vi "ADC.vi"() -> ()   [LabVIEW 2013]
uses:
  <vilib>/Utility/file.llb/Write To Spreadsheet File (DBL).vi
panel:
  out "Відповідне значення температури з урахуванням коеф. А":dbl
  in  "А коеф.":dbl=0.00784
  out "I А":dbl
  out "Rx оМ з урахуванням\n томпер. коеф А.":dbl
  out "Rx оМ":dbl
  out "Uadc В":dbl
  in  "А коеф.":dbl=0.0079
  in  "Path":path=path "C:/Temp_Do_msp430g2231/USB_PC_Config/first.csv"
  out "Відповідне значення температури":dbl
  in  "Опір при температурі ххС":dbl=1000.0
  in  "Значення Т ххС":dbl=25.0
  in  "АЦП розрядність":dbl=1024.0
  in  "Vcc":dbl=3.3
  in  "R0":dbl=1200.0
  out "Thermometer":dbl(slide) scale=-55.0..155.0
  out "Посилка":i32
  in  "stop":bool
  out "відповідний Числовий тип":dbl
  out "Отриманий текст":string
  in  "Вибір порта для\n отримання даних":refnum<visa-resource-name>
  # "Налаштування  для  датчика"
  # "Отримані дані"
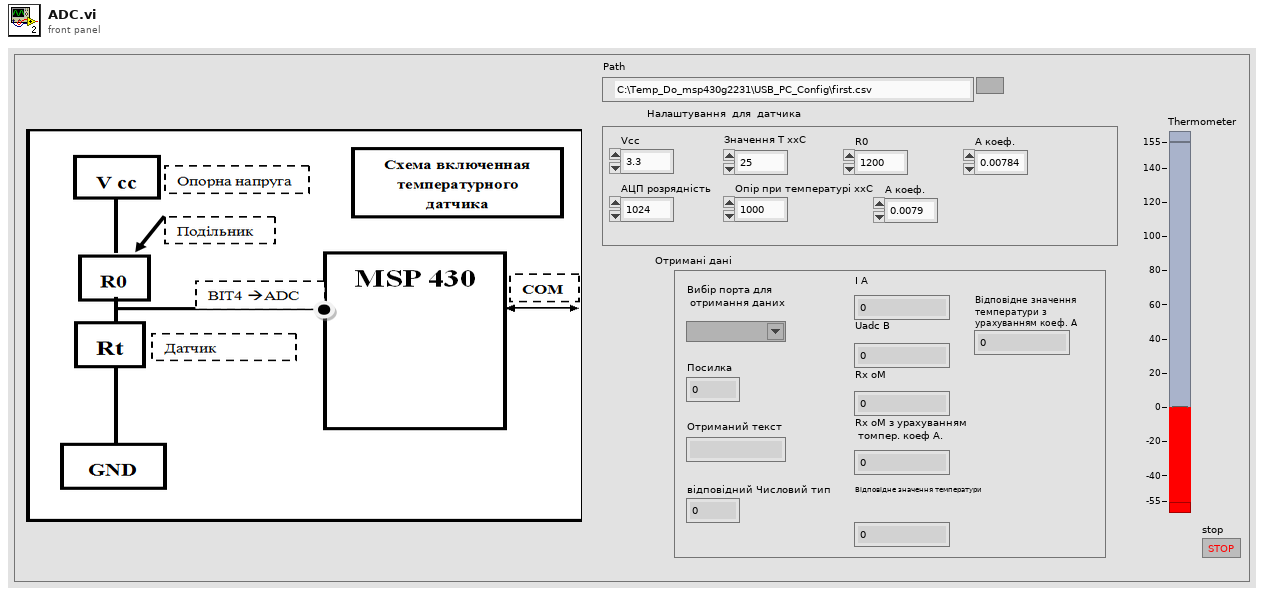
[diagram p1: front panel]
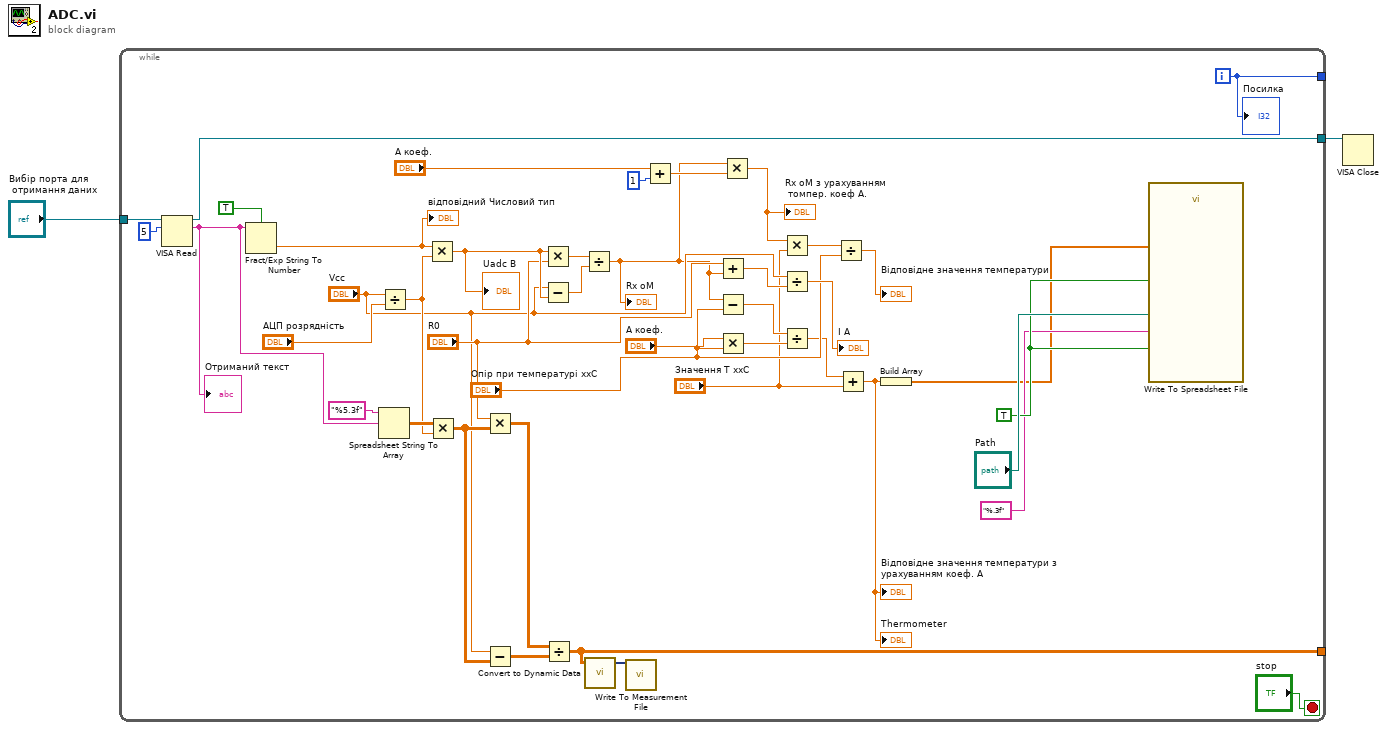
[diagram p0: block diagram]
diagram:
  n1 = while {
    tunnel: "Вибір порта для\n отримання даних" -> [w44]
    tunnel: [w25] -> _
    tunnel: [w28] -> _
    tunnel: [w32] -> w1
    i -> [w25]
    stop <- "stop" stop-if-true
    w27 = TRUE
    n2 = VISA Read(VISA resource name=w44, byte count=u32 5) -> (VISA resource name out=w32:refnum<visa-resource-name>, read buffer=w40:string)  [unwired: 1 in, 2 out]
    "Отриманий текст" <- w40
    n3 = Fract/Exp String To Number(use system decimal point (T)=TRUE, string=w40) -> (number=w33:dbl)  [unwired: 2 in, 1 out]
    "відповідний Числовий тип" <- w33
    n4 = Spreadsheet String To Array(format string="%5.3f", spreadsheet string=w40) -> (array=w34:dbl[][])  [unwired: 2 in]
    n5 = Divide(x="Vcc", y="АЦП розрядність") -> (x/y=w30:dbl)
    n6 = Multiply(x=w33, y=w30) -> (x*y=w19:dbl)
    "Uadc В" <- w19
    n7 = Multiply(x=w34, y=w30) -> (x*y=w39:dbl[][])
    n8 = Multiply(x="R0", y=w39) -> (x*y=w38:dbl[][])
    n9 = Subtract(x="Vcc", y=w39) -> (x-y=w37:dbl[][])
    n10 = Multiply(x=w19, y="R0") -> (x*y=w20:dbl)
    n11 = Subtract(x="Vcc", y=w19) -> (x-y=w21:dbl)
    n12 = Divide(x=w38, y=w37) -> (x/y=w28:dbl[][])
    n13 = Divide(x=w20, y=w21) -> (x/y=w10:dbl)
    "Rx оМ" <- w10
    n14 = call "Convert to Dynamic Data"("2D Array"=w28) -> ("Dynamic Data Type"=w35:dynamicdata)  [unwired: 3 in]
    n15 = call "Write To Measurement File"("Signals"=w35) -> ()  [unwired: 16 in, 3 out]
    n16 = Add(x="А коеф.", y=1) -> (x+y=w18:dbl)
    n17 = Add(x="R0", y=w10) -> (x+y=w16:dbl)
    n18 = Subtract(x=w10, y="Опір при температурі ххС") -> (x-y=w7:dbl)
    n19 = Multiply(x="А коеф.", y="Опір при температурі ххС") -> (x*y=w6:dbl)
    n20 = Multiply(x=w10, y=w18) -> (x*y=w13:dbl)
    "Rx оМ з урахуванням\n томпер. коеф А." <- w13
    n21 = Multiply(x=w13, y="Значення Т ххС") -> (x*y=w12:dbl)
    n22 = Divide(x="Vcc", y=w16) -> (x/y=→"I А":dbl)
    n23 = Divide(x=w7, y=w6) -> (x/y=w5:dbl)
    n24 = Divide(x=w12, y="Опір при температурі ххС") -> (x/y=→"Відповідне значення температури":dbl)
    n25 = Add(x=w5, y="Значення Т ххС") -> (x+y=w3:dbl)
    "Thermometer" <- w3
    "Відповідне значення температури з урахуванням коеф. А" <- w3
    n26 = Build Array "Build Array"(w3) -> (w24:dbl[])
    n27 = call-poly <vilib>:"Write To Spreadsheet File.vi"("transpose? (no:F)"=w27, "format (%.3f)"="%.3f", "append to file? (new file:F)"=w27, "1D data"=w24, "file path (dialog if empty)"="Path") -> ()  [unwired: 3 in, 1 out]
    "Посилка" <- w25
  }
  n28 = VISA Close(VISA resource name=w1) -> ()  [unwired: 1 in, 1 out]
